vi "Read Data Access.vi"(8 "error in (no error)":errorcluster, 11 "Process in":refnum<class "Process.lvclass">) -> (0 "error out":errorcluster, 2 "Data Access":refnum<class "Data Access Engine (Express).lvclass">, 3 "Process out":refnum<class "Process.lvclass">)   [LabVIEW 2027, in "VS Inline Async API (Express).lvlib" / "Process.lvclass"]
uses:
  Process.lvclass
  _Data Access Engine (Express)/Data Access Engine (Express)/Data Access Engine (Express).lvclass
  Process.lvclass/Process.ctl
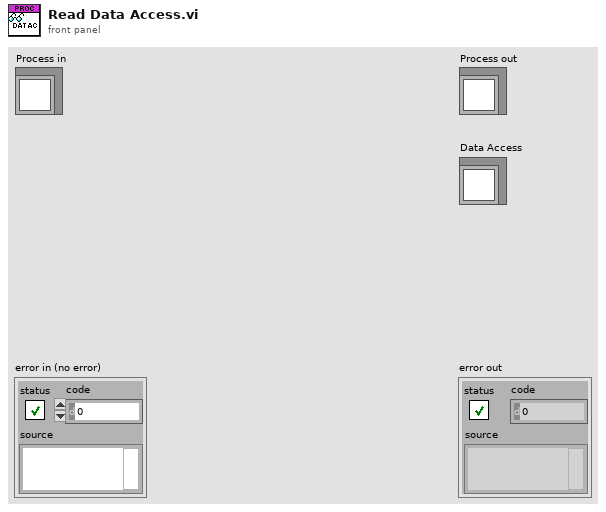
[diagram p1: front panel]
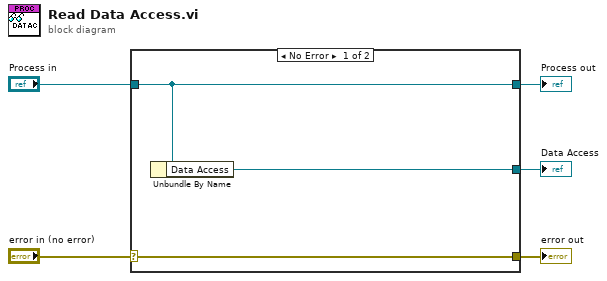
[diagram p0: block diagram]
diagram:
  n1 = case shown="No Error" "error in (no error)" {
    selector: "error in (no error)" -> [w8 w9]
    tunnel: [w8 w9] -> w4
    tunnel: [w7 w10] -> w2
    tunnel: "Process in" -> [w7 w10]
    tunnel: [w6 _] -> w1
    frame No Error {
      n2 = Unbundle By Name(w7) -> ("Data Access"=w6:refnum<class "Data Access Engine (Express).lvclass">)
    }
    frame Error {
    }
  }
  "error out" <- w4
  "Process out" <- w2
  "Data Access" <- w1
